vi "Config file functional global modes.vi"(0 "File path":path, 1 "Mode":T1, 5 "refnum in":refnum<file>, 7 "text to write":string, 11 "error in":errorcluster) -> (4 "file path out":path, 6 "refnum out":refnum<file>, 8 "text in file":string, 15 "error out":errorcluster)   [LabVIEW 2010]
doc: "This .vi executes the actions on the Quartz config files which store the information on status of the front panel controls. On startup, these config files populate the front panel controls.\n\nActions :\n<B>Set Filepath</B> - Opens a file ref to the input file or creates a config file (flattenned array of variants) if the file does not exist.\n<B>Read File</B> - Returns all of the text of the input fille.\n<B>Rewrite file</B> - Writes the input text to the file."
uses:
  HHMI - Config file functional global mode enum.ctl
panel:
  out "size (in bytes)":i64
  out "length":i32
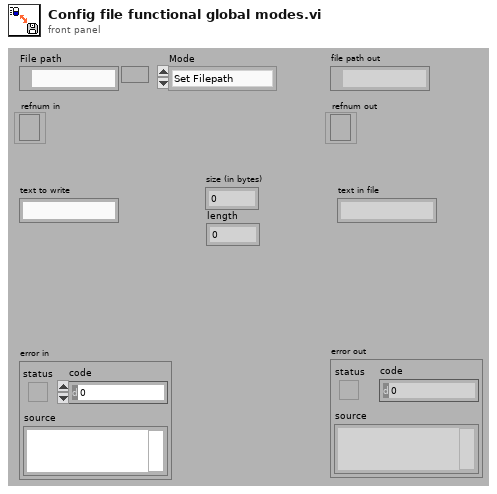
[diagram p1: front panel]
types:
  T1 = typedef "HHMI - Config file functional global mode enum.ctl" = enum16{"Set Filepath", "Read file", "Rewrite file"}
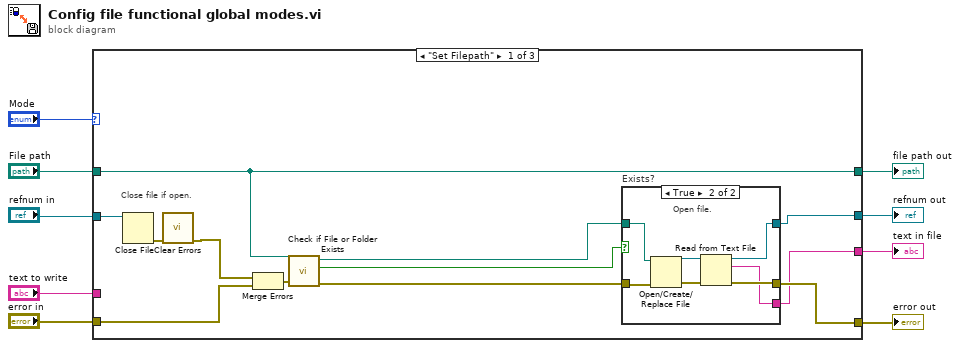
[diagram p0: block diagram]
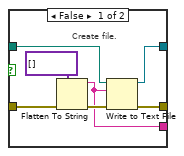
[diagram p2: hidden frame]
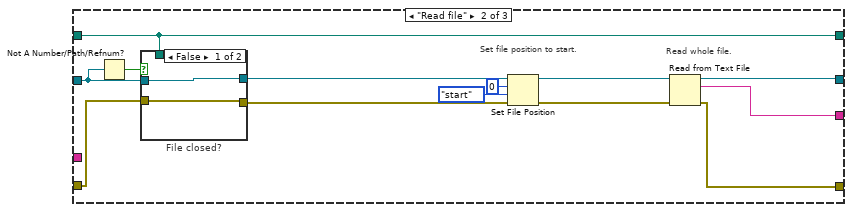
[diagram p3: hidden frame]
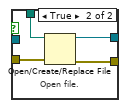
[diagram p4: hidden frame]
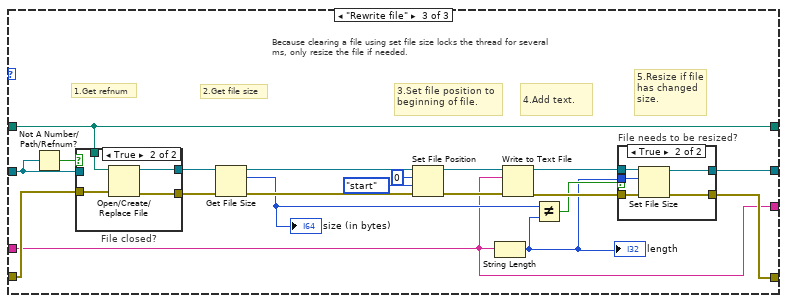
[diagram p5: hidden frame]
diagram:
  n1 = case shown="\"Set Filepath\"" "Mode" {
    tunnel: [w13 w38 w60] -> w3
    tunnel: [w17 w47 w65] -> w4
    tunnel: "error in" -> [w12 w42 w62]
    tunnel: [w18 w48 w69] -> w6
    tunnel: "refnum in" -> [w15 w39 w61]
    tunnel: "File path" -> [w13 w38 w60]
    tunnel: "text to write" -> [_ _ w55]
    tunnel: [w16 w44 w55] -> w9
    frame "Set Filepath" {
      # "Close file if open."
      n2 = Close File(refnum=w15) -> (error out=w14:errorcluster)  [unwired: 1 in, 1 out]
      n3 = call <vilib>:"Clear Errors.vi"("error in (no error)"=w14) -> ("error out"=w10:errorcluster)  [unwired: 6 out]
      n4 = Merge Errors(w10, w12) -> (w11:errorcluster)
      n5 = call <vilib>:"Check if File or Folder Exists.vi"("error in (no error)"=w11, "path"=w13) -> ("error out"=w20:errorcluster, "file or folder exists?"=w19:bool, "dup path"=w21:path)  [unwired: 7 out]
      n6 = case "Exists?" shown="True" w19 {
        tunnel: w21 -> [w26 w34]
        tunnel: w20 -> [w24 w35]
        tunnel: [w28 w31] -> w17
        tunnel: [w27 w33] -> w18
        tunnel: [w22 w29] -> w16
        frame False {
          # "Create file."
          n7 = Flatten To String(anything=variant[] [], error in (no error)=w24) -> (data string=w22:string, error out=w25:errorcluster)  [unwired: 3 out]
          n8 = Write to Text File(file (use dialog)=w26, text=w22, error in=w25) -> (refnum out=w28:refnum<file>, error out=w27:errorcluster)  [unwired: 2 out]
        }
        frame True {
          # "Open file."
          n9 = Open/Create/Replace File(file path (use dialog)=w34, error in=w35) -> (refnum out=w30:refnum<file>, error out=w32:errorcluster)  [unwired: 5 out]
          n10 = Read from Text File(file (use dialog)=w30, error in=w32) -> (refnum out=w31:refnum<file>, text=w29:string, error out=w33:errorcluster)  [unwired: 3 out]
        }
      }
    }
    frame "Read file" {
      # "Read whole file."
      # "Set file position to start."
      n11 = Not A Number/Path/Refnum?(number/path/refnum=w39) -> (NaN/Path/Refnum?=w43:bool)
      n12 = case "File closed?" shown="False" w43 {
        tunnel: w42 -> [w49 w54]
        tunnel: w39 -> [w50 _]
        tunnel: w38 -> [_ w53]
        tunnel: [w49 w52] -> w41
        tunnel: [w50 w51] -> w40
        frame False {
        }
        frame True {
          # "Open file."
          n13 = Open/Create/Replace File(file path (use dialog)=w53, error in=w54) -> (refnum out=w51:refnum<file>, error out=w52:errorcluster)  [unwired: 5 out]
        }
      }
      n14 = Set File Position(offset (in bytes) (0)=i64 0, refnum=w40, from (0:start)=enum16{"start", "end", "current"}."start", error in=w41) -> (refnum out=w46:refnum<file>, error out=w45:errorcluster)
      n15 = Read from Text File(file (use dialog)=w46, error in=w45) -> (refnum out=w47:refnum<file>, text=w44:string, error out=w48:errorcluster)  [unwired: 3 out]
    }
    frame "Rewrite file" {
      # "5.Resize if file has changed size."
      # "4.Add text."
      # "3.Set file position to beginning of file."
      # "2.Get file size"
      # "1.Get refnum"
      # "Because clearing a file using set file size locks the thread for several\nms, only resize the file if needed."
      n16 = Not A Number/Path/Refnum?(number/path/refnum=w61) -> (NaN/Path/Refnum?=w63:bool)
      n17 = case "File closed?" shown="True" w63 {
        tunnel: w62 -> [w75 w80]
        tunnel: w61 -> [w76 _]
        tunnel: w60 -> [_ w79]
        tunnel: [w75 w78] -> w59
        tunnel: [w76 w77] -> w58
        frame False {
        }
        frame True {
          n18 = Open/Create/Replace File(file path (use dialog)=w79, error in=w80) -> (refnum out=w77:refnum<file>, error out=w78:errorcluster)  [unwired: 5 out]
        }
      }
      n19 = Get File Size(file=w58, error in=w59) -> (refnum out=w73:refnum<file>, size (in bytes)=w70:i64, 0:w74:errorcluster)
      "size (in bytes)" <- w70
      n20 = Set File Position(offset (in bytes) (0)=i64 0, refnum=w73, from (0:start)=enum16{"start", "end", "current"}."start", error in=w74) -> (refnum out=w72:refnum<file>, error out=w71:errorcluster)
      n21 = String Length(string=w55) -> (length=w64:i32)
      "length" <- w64
      n22 = Write to Text File(file (use dialog)=w72, text=w55, error in=w71) -> (refnum out=w67:refnum<file>, error out=w68:errorcluster)  [unwired: 2 out]
      n23 = Not Equal?(x=w70, y=w64) -> (x != y?=w66:bool)
      n24 = case "File needs to be resized?" shown="True" w66 {
        tunnel: [w82 w87] -> w69
        tunnel: w68 -> [w82 w86]
        tunnel: w67 -> [w81 w85]
        tunnel: [w81 w84] -> w65
        tunnel: w64 -> [_ w83]
        frame False {
        }
        frame True {
          n25 = Set File Size(4:w86, 6:w83, 7:w85) -> (0:w87:errorcluster, 3:w84:refnum<file>)
        }
      }
    }
  }
  "text in file" <- w9
  "error out" <- w6
  "refnum out" <- w4
  "file path out" <- w3
